vi "Tabor 5064 - Setup Standard Waveforms (SubVI).vi"(0 "amps (V)":dbl[](array[numeric]), 1 "waveform_type":u16(ring)=1 items=["DC", "Sine", "Triangle", "Square"], 2 "GPIB Address":string, 5 "offsets (V)":dbl[](array[numeric]), 7 "freq":dbl, 9 "phases (deg)":dbl[](array[numeric]), 11 "error_in":errorcluster, 12 "write_delay (ms)":u32=100) -> (15 "error_out":errorcluster)   [LabVIEW 2018]
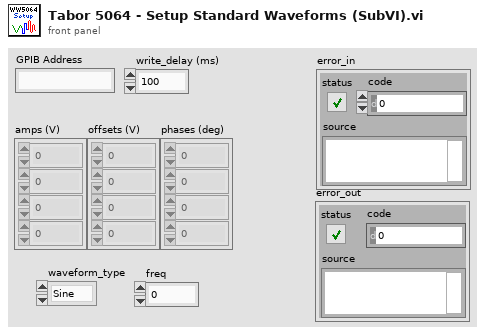
[diagram p1: front panel]
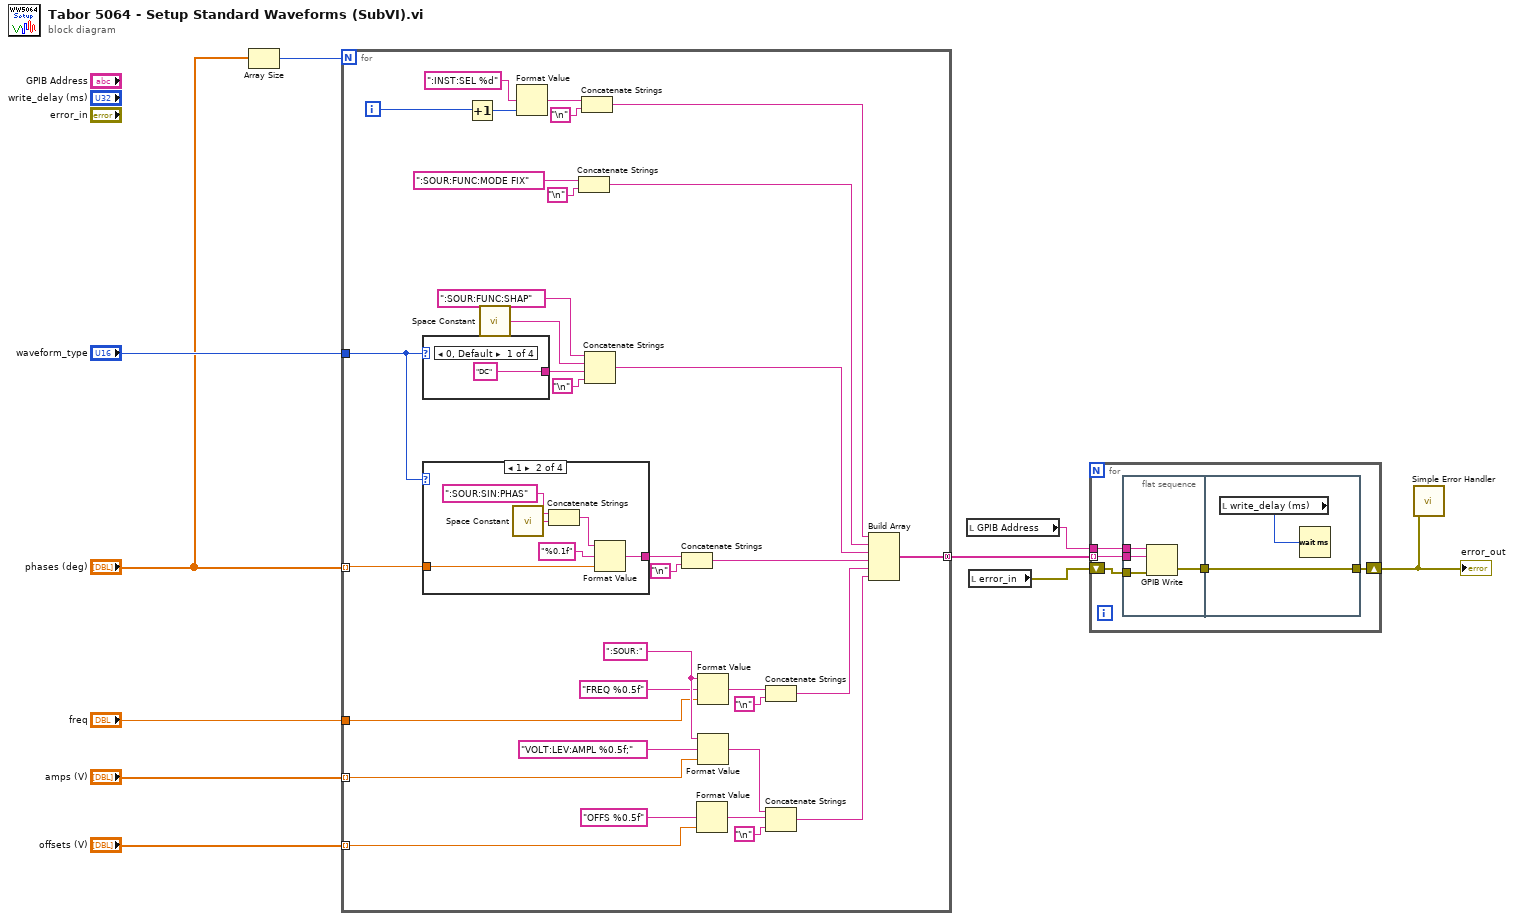
[diagram p0: block diagram]
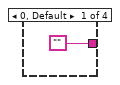
[diagram p2: hidden frame]
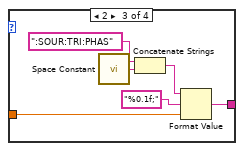
[diagram p3: hidden frame]
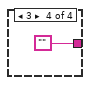
[diagram p4: hidden frame]
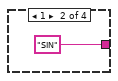
[diagram p5: hidden frame]
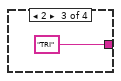
[diagram p6: hidden frame]
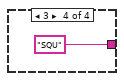
[diagram p7: hidden frame]
diagram:
  n1 = Array Size(array="phases (deg)") -> (size(s)=w8:i32)
  n2 = for {
    N: w8 -> [_]
    tunnel: "freq" -> [w40]
    tunnel: "waveform_type" -> [w36]
    tunnel: "phases (deg)" -> [w32] mode=indexing
    tunnel: "amps (V)" -> [w31] mode=indexing
    tunnel: "offsets (V)" -> [w30] mode=indexing
    tunnel: [w17] -> w4 mode=concatenating
    i -> [w33]
    w44 = ":SOUR:"
    n3 = case shown="0, Default" w36 {
      tunnel: ["DC" "SIN" "TRI" "SQU"] -> w37
      frame 0, Default {
      }
      frame 1 {
      }
      frame 2 {
      }
      frame 3 {
      }
    }
    n4 = case shown="1" w36 {
      tunnel: w32 -> [_ w47 w55 _]
      tunnel: ["" w46 w52 ""] -> w24
      frame 0, Default {
      }
      frame 1 {
        n5 = call <vilib>:"Space Constant.vi"() -> ("String"=w50:string)
        n6 = Concatenate Strings(":SOUR:SIN:PHAS", w50) -> (w48:string)
        n7 = Format Value(string ("")=w48, format string="%0.1f", value (0)=w47) -> (output string=w46:string)
      }
      frame 2 {
        n8 = call <vilib>:"Space Constant.vi"() -> ("String"=w56:string)
        n9 = Concatenate Strings(":SOUR:TRI:PHAS", w56) -> (w53:string)
        n10 = Format Value(string ("")=w53, format string="%0.1f;", value (0)=w55) -> (output string=w52:string)
      }
      frame 3 {
      }
    }
    n11 = Increment(x=w33) -> (x+1=w34:i32)
    n12 = call <vilib>:"Space Constant.vi"() -> ("String"=w38:string)
    n13 = Format Value(format string=":INST:SEL %d", value (0)=w34) -> (output string=w25:string)  [unwired: 1 in]
    n14 = Concatenate Strings(":SOUR:FUNC:MODE FIX", "\n") -> (w12:string)
    n15 = Concatenate Strings(w25, "\n") -> (w11:string)
    n16 = Concatenate Strings(":SOUR:FUNC:SHAP", w38, w37, "\n") -> (w15:string)
    n17 = Concatenate Strings(w24, "\n") -> (w20:string)
    n18 = Format Value(format string="OFFS %0.5f", value (0)=w30) -> (output string=w22:string)  [unwired: 1 in]
    n19 = Format Value(string ("")=w44, format string="FREQ %0.5f", value (0)=w40) -> (output string=w23:string)
    n20 = Format Value(string ("")=w44, format string="VOLT:LEV:AMPL %0.5f;", value (0)=w31) -> (output string=w21:string)
    n21 = Concatenate Strings(w23, "\n") -> (w19:string)
    n22 = Concatenate Strings(w21, w22, "\n") -> (w18:string)
    n23 = Build Array(w11, w12, w15, w20, w19, w18) -> (w17:string[])
  }
  n24 = local read "GPIB Address"() -> (w3:string)
  n25 = local read "error_in"() -> (w1:errorcluster)
  n26 = for {
    tunnel: w3 -> [w67]
    tunnel: w4 -> [w66] mode=indexing
    shift-right: [w65] -> w2
    shift-left: w1 -> [w64]
    n27 = flat-sequence {
      tunnel: w67 -> [w71]
      tunnel: w66 -> [w70]
      tunnel: w64 -> [w68]
      tunnel: [w69] -> w63
      tunnel: [w73] -> w65
      tunnel: w63 -> [w73]
      frame #0 {
        n28 = GPIB Write(0:w71, 1:w70, 3:w68) -> (6:w69:errorcluster)  [unwired: 2 in, 1 out]
      }
      frame #1 {
        n29 = local read "write_delay (ms)"() -> (w72:u32)
        n30 = Wait (ms)(milliseconds to wait=w72) -> ()  [unwired: 1 out]
      }
    }
  }
  "error_out" <- w2
  n31 = call <vilib>:"Simple Error Handler.vi"("error in (no error)"=w2) -> ()  [unwired: 4 in, 5 out]
